vi "PH_4_Pos_Selector.PC Write PSDB.vi"(0 "i ref in":refnum<vi>, 5 "error IO":errorcluster) -> (14 "i ref out":refnum<vi>, 19 "error out":errorcluster)   [LabVIEW 2014, in "PH_4_Pos_Selector.lvlib"]
doc: "This is the proc case which writes data to the PHELIX shot data base."
uses:
  PH_4_Pos_Selector.lvlib
  PH_4_Pos_Selector.Position Selector.ctl
  PH_PSDBWriter/PH_PSDBWriter.Numeric dataset.ctl
  PH_PSDBWriter/PH_PSDBWriter.lvlib
  PH_AxisGUI_BaseClass/PH_AxisGUI_BaseClass.lvlib
panel:
  in  "Current Position":T1 items=["unknown", "Position I", "Position II", "Position III", "Position IV", "moving"]
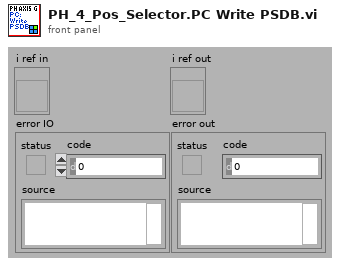
[diagram p1: front panel]
types:
  T1 = typedef "PH_4_Pos_Selector.lvlib/PH_4_Pos_Selector.Position Selector.ctl" = u16
  T2 = typedef "PH_PSDBWriter.lvlib/PH_PSDBWriter.Numeric dataset.ctl" = cluster{"name":string, "data":dbl, "unit":string}
  T3 = typedef "PH_4_Pos_Selector.lvlib/PH_4_Pos_Selector.i attribute.ctl" = cluster{"GUI Refs":cluster{"Position I":refnum<vi>, "Position II":refnum<vi>, "Position III":refnum<vi>, "Position IV":refnum<vi>, "rel. Mode?":refnum<vi>, "Define Selector":refnum<vi>}, "Current Position":T1, "Service ID Position":i32, "Position Array":T4[], "Description Array":string[], "relative Mode":bool, "Wanted Define Selector Position":string}
  T4 = typedef "PH_4_Pos_Selector.lvlib/PH_4_Pos_Selector.Position.ctl" = cluster{"Axis 1":dbl, "Axis 2":dbl}
  T5 = typedef "PH_AxisGUI_BaseClass.lvlib/PH_AxisGUI_BaseClass.i attribute.ctl" = cluster{"Axes":T6[]}
  T6 = typedef "PH_AxisGUI_BaseClass.lvlib/PH_AxisGUI_BaseClass.Axis Attributes.ctl" = cluster{"Axis GUI Refs":T7, "Address":T8, "Name":string, "Label \"Back\"":string, "Labell \"Forth\"":string, "Moving?":bool}
  T7 = typedef "PH_AxisGUI_BaseClass.lvlib/PH_AxisGUI_BaseClass.Axis GUI Refs.ctl" = cluster{"Back":refnum<vi>, "Forth":refnum<vi>, "Status":refnum<vi>, "Target":refnum<vi>, "Address":refnum<vi>, "Status Bar":refnum<vi>, "Settings":refnum<vi>, "Activity":refnum<vi>, "Clear Error":refnum<vi>}
  T8 = typedef "PH_Stepmotor_BaseClass.lvlib/PH_Stepmotor_BaseClass.Axis Address.ctl" = cluster{"Instance":string, "Motor Nr":i32}
  T9 = typedef "PH_Stepmotor_BaseClass.lvlib/PH_Stepmotor_BaseClass.Axis Settings.ctl" = cluster{"Sign change":bool, "Width":dbl, "Calibration":dbl, "Unit":string, "Motor Type":T10, "Unit Width":string, "Unit CF":string}
  T10 = typedef "PH_Stepmotor_BaseClass.lvlib/PH_Stepmotor_BaseClass.Motor Type.ctl" = enum16{"Unspecific", "OWIS 49.120.2633", "OWIS 49.060.1033", "OWIS 43.040.2558", "Diamond Motion 2200 series", "OWIS 49.120.266B.MV6", "Calorimeter", "Linear Stage 1", "MICOS VT-80", "MICOS VT-80 S", "Standa Rotstage nt0.95A", "PUF RA 320.200", "PUF RA 800.200", "PUF RA 800.400", "PUF RA 400.50", "1324.nn.800.50", "1324.n9c.800.50", "1324.nn.320.200", "1324.nn.400.200", "1324.nn.800.200", "1324.nn.400.50", "1324.8c9c.800.50", "1324.8c9c.400.200"}
  T11 = typedef "PH_PSDBWriter.lvlib/PH_PSDBWriter.String dataset.ctl" = cluster{"name":string, "data":string, "unit":string}
  T12 = typedef "PH_PSDBWriter.lvlib/PH_PSDBWriter.PSDB Dataset.ctl" = cluster{"Version":i32, "2D data Input":T13[], "Boolean Input":T15[], "Image Input":T16[], "Numeric Input":T2[], "String Input":T11[]}
  T13 = typedef "PH_PSDBWriter.lvlib/PH_PSDBWriter.2D dataset.ctl" = cluster{"name":string, "data":dbl[][], "axis description":T14}
  T14 = typedef "PSDB.lvlib/PSDB_AxisDescription.ctl" = cluster{"x axis label":string, "y axis label":string, "x axis unit":string, "y axis unit":string}
  T15 = typedef "PH_PSDBWriter.lvlib/PH_PSDBWriter.Boolean dataset.ctl" = cluster{"name":string, "data":bool, "unit":string}
  T16 = typedef "PH_PSDBWriter.lvlib/PH_PSDBWriter.Image dataset.ctl" = cluster{"name":string, "data":T17, "unit":string}
  T17 = typedef "IMAQ Image.ctl" = refnum<image>
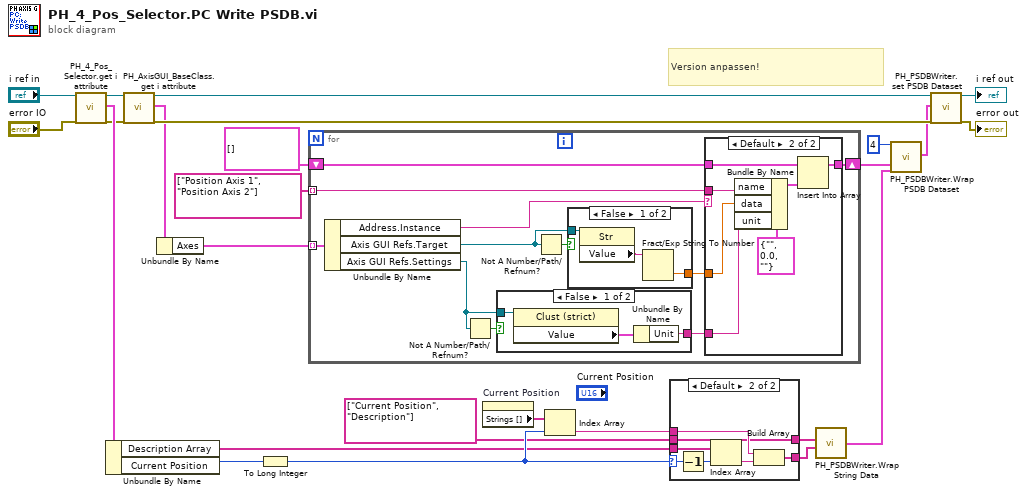
[diagram p0: block diagram]
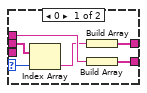
[diagram p2: hidden frame]
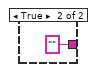
[diagram p3: hidden frame]
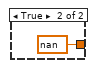
[diagram p4: hidden frame]
diagram:
  # "Version anpassen!"
  n1 = call "PH_4_Pos_Selector.get i attribute.vi"("i ref in"="i ref in", "error in (no error)"="error IO") -> ("i ref out"=w3:refnum<vi>, "i attribute"=w25:T3, "error out"=w2:errorcluster)  [unwired: 15 in]
  n2 = Unbundle By Name(w25) -> ("Description Array"=w1:string[], "Current Position"=w23:T1)
  n3 = call "PH_AxisGUI_BaseClass.get i attribute.vi"("i ref in"=w3, "error in (no error)"=w2) -> ("i ref out"=w15:refnum<vi>, "i attribute"=w18:T5, "error out"=w19:errorcluster)  [unwired: 15 in]
  n4 = Unbundle By Name(w18) -> ("Axes"=w6:T6[])
  n5 = To Long Integer(number=w23) -> (32bit integer=w21:i32)
  n6 = for {
    tunnel: string[] ["Position Axis 1", "Position Axis 2"] -> [w36] mode=indexing
    shift-right: [w35] -> w9
    shift-left: T2[] [] -> [w34]
    tunnel: w6 -> [w33] mode=indexing
    n7 = Unbundle By Name(w33) -> ("Address.Instance"=w32:string, "Axis GUI Refs.Target"=w28:refnum<vi>, "Axis GUI Refs.Settings"=w27:refnum<vi>)
    n8 = Not A Number/Path/Refnum?(number/path/refnum=w27) -> (NaN/Path/Refnum?=w26:bool)
    n9 = case shown="False" w26 {
      tunnel: w27 -> [w39 _]
      tunnel: [w37 "" ("Unit")] -> w30
      frame False {
        n10 = property class="Clust (strict)"(reference=w39) -> ("Value"=w38:T9)  [unwired: 1 in, 2 out]
        n11 = Unbundle By Name(w38) -> ("Unit"=w37:string)
      }
      frame True {
      }
    }
    n12 = Not A Number/Path/Refnum?(number/path/refnum=w28) -> (NaN/Path/Refnum?=w29:bool)
    n13 = case shown="False" w29 {
      tunnel: w28 -> [w43 _]
      tunnel: [w41 nan] -> w31
      frame False {
        n14 = property class="Str"(reference=w43) -> ("Value"=w42:string)  [unwired: 1 in, 2 out]
        n15 = Fract/Exp String To Number(string=w42) -> (number=w41:dbl)  [unwired: 3 in, 1 out]
      }
      frame True {
      }
    }
    n16 = case shown="Default" w32 {
      tunnel: w36 -> [_ w52]
      tunnel: w31 -> [_ w51]
      tunnel: w30 -> [_ w50]
      tunnel: [w45 w48] -> w35
      tunnel: w34 -> [w45 w47]
      frame "", "N/A" {
      }
      frame Default {
        n17 = Bundle By Name(cluster=T2 {"name"="", "data"=0.0, "unit"=""} ("Numeric data"), "name"=w52, "data"=w51, "unit"=w50) -> (w49:T2)
        n18 = Insert Into Array(array=w47, new element=w49) -> (w48:T2[])  [unwired: 1 in]
      }
    }
  }
  n19 = property on="Current Position" class="Ring (strict)"() -> ("Strings []"=w24:string[])  [unwired: 2 in, 2 out]
  n20 = Index Array(array=w24, index=w21) -> (element=w22:string)
  n21 = case shown="Default" w21 {
    selector: w21 -> [w56 w60]
    tunnel: [w53 w59] -> w11
    tunnel: w22 -> [w58 w65]
    tunnel: [w57 w64] -> w12
    tunnel: w1 -> [_ w63]
    tunnel: string[] ["Current Position", "Description"] -> [w55 w59]
    frame 0 {
      n22 = Index Array(array=w55, index=w56) -> (element=w54:string)
      n23 = Build Array(w54) -> (w53:string[])
      n24 = Build Array(w58) -> (w57:string[])
    }
    frame Default {
      n25 = Decrement(x=w60) -> (x-1=w61:i32)
      n26 = Index Array(array=w63, index=w61) -> (element=w62:string)
      n27 = Build Array(w65, w62) -> (w64:string[])
    }
  }
  n28 = call "PH_PSDBWriter.Wrap String Data.vi"("Data Array"=w12, "Name Array"=w11) -> ("PSDB String Data Array"=w10:T11[])  [unwired: 2 in]
  n29 = call "PH_PSDBWriter.Wrap PSDB Dataset.vi"("Version"=4, "Numeric Input"=w9, "String Input"=w10) -> ("PSDB Dataset"=w8:T12)  [unwired: 16 in]
  n30 = call "PH_PSDBWriter.set PSDB Dataset.vi"("VI in"=w15, "PSDB Dataset"=w8, "error in (no error)"=w19) -> ("VI out"=→"i ref out":refnum<vi>, "error out"=→"error out":errorcluster)  [unwired: 15 in]
